vi "Obtain Message Queue.vi"(7 "max queue size (-1, unlimited)":i32=-1, 8 "error in (no error)":errorcluster, 11 "Queue name":string) -> (0 "error out":errorcluster, 3 "Message Queue":refnum<queue>)   [LabVIEW 2017]
doc: "Create a queue with the Message Cluster data type."
uses:
  Typedefs/Message Cluster.ctl
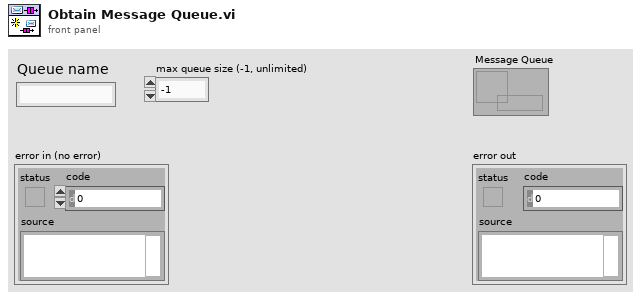
[diagram p1: front panel]
types:
  T1 = typedef "Message Cluster.ctl" = cluster{"Message":string, "Message Data":variant}
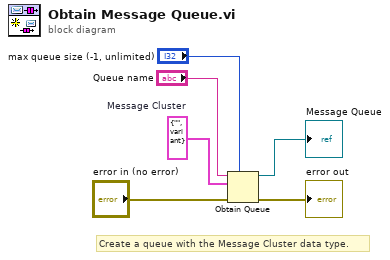
[diagram p0: block diagram]
diagram:
  w6 = T1 {"Message"="", "Message Data"=variant}  # Message Cluster
  # "Create a queue with the Message Cluster data type."
  n1 = Obtain Queue(max queue size (-1, unlimited)="max queue size (-1, unlimited)", name (unnamed)="Queue name", element data type=w6, error in (no error)="error in (no error)") -> (queue out=→"Message Queue":refnum<queue>, error out=→"error out":errorcluster)  [unwired: 1 in, 1 out]
